vi "SetAttributes.vi"(8 "error in (no error)":errorcluster, 10 "Payload":cluster{"Name":string, "Value":bool}, 11 "Set by Name Msg in":refnum<class "Set by Name Msg.lvclass">) -> (0 "error out":errorcluster, 3 "Set by Name Msg out":refnum<class "Set by Name Msg.lvclass">)   [LabVIEW 2019, in "DIG_IO.lvlib" / "Set by Name Msg.lvclass"]
uses:
  Set by Name Msg.lvclass
  Set by Name Msg.lvclass/Set by Name Msg.ctl
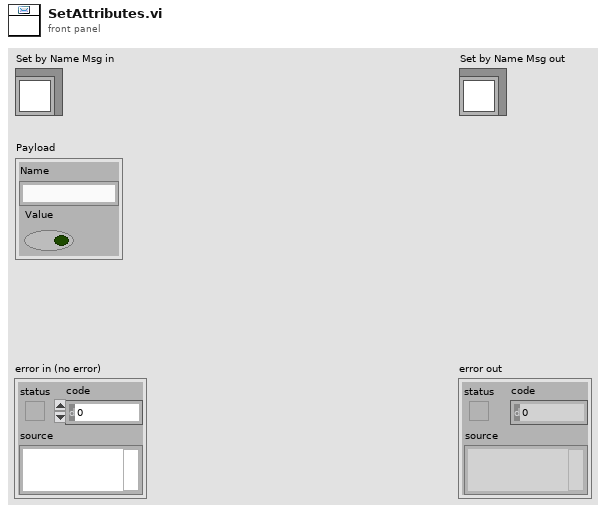
[diagram p1: front panel]
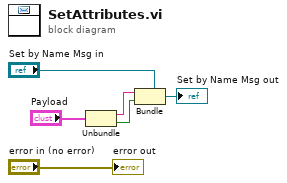
[diagram p0: block diagram]
diagram:
  n1 = Unbundle("Payload") -> ("Name"=w2:string, "Value"=w1:bool)
  n2 = Bundle(cluster="Set by Name Msg in", w2, w1) -> (→"Set by Name Msg out":refnum<class "Set by Name Msg.lvclass">)
  "error out" <- "error in (no error)"
